vi "WriteImageFileARGB.vi"(8 "error in (no error)":errorcluster, 10 "Filepath":path, 11 "ARGB Image Source":refnum<data-value>) -> (0 "error out":errorcluster, 3 "Filepath (duplicate)":path)   [LabVIEW 2020, in "g_ar_toolkit.image.lvlib"]
uses:
  g_ar_toolkit.image.lvlib
  g_ar_toolkit.common/Module Path.vi
  <vilib>/Utility/error.llb/Error Cluster From Error Code.vi
  9723f547-2605-4a38-b7b5-a8bc0a93fff0.vi
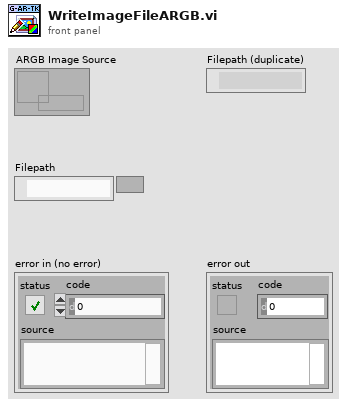
[diagram p1: front panel]
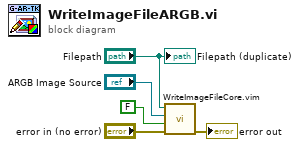
[diagram p0: block diagram]
diagram:
  n1 = call "WriteImageFileCore.vim"("error in (no error)"="error in (no error)", "SaveAlpha"=FALSE, "Src"="ARGB Image Source", "Filepath"="Filepath") -> ("error out"=→"error out":errorcluster)  [unwired: 7 in]
  "Filepath (duplicate)" <- "Filepath"
